vi "FABR-What Now.vi"(0 "Runtime in":T1, 2 "Queue in":refnum<queue>, 7 "SCL in":cluster{T3[]}[](array[cluster]), 11 "error in (no error)":errorcluster) -> (4 "Runtime thru":T1, 8 "SCL thru":cluster{T3[]}[](array[cluster]), 15 "error out":errorcluster)   [LabVIEW 2020]
uses:
  Typedefs/FABR-Stimulus Condition.ctl
  Typedefs/FABR-Runtime Data.ctl
  Typedefs/FABR-Stimulus Ticket.ctl
  Typedefs/FABR-Queue Data.ctl
  Typedefs/FABR-Parameters.ctl
  Typedefs/FABR-Stimulus.ctl
  Typedefs/FABR-Sequence.ctl
  Typedefs/FABR-Order.ctl
  Typedefs/FABR-Response.ctl
  Threshold Estimation VIs/ABR3-Threshold Estimation Parameters.ctl
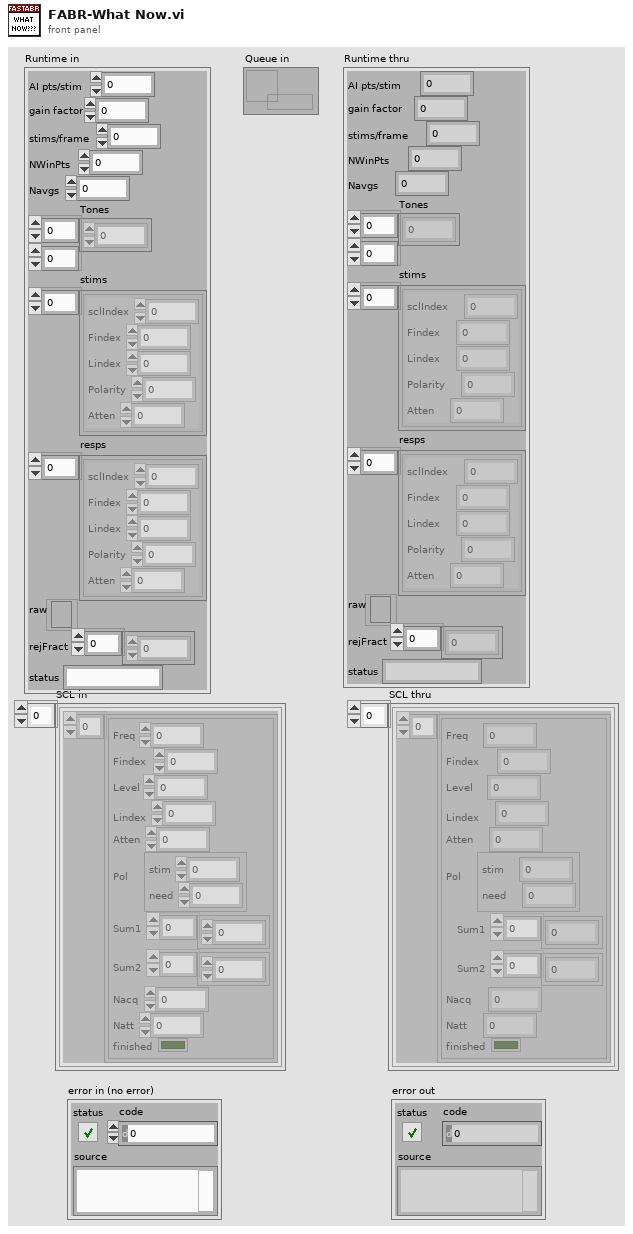
[diagram p1: front panel]
types:
  T1 = typedef "FABR-Runtime Data.ctl" = cluster{"AI pts/stim":i32, "gain factor":dbl, "stims/frame":i32, "NWinPts":i32, "Navgs":i32, "Tones":dbl[][], "stims":T2[], "resps":T2[], "raw":refnum<file>, "rejFract":dbl[], "status":string}
  T2 = typedef "FABR-Stimulus Ticket.ctl" = cluster{"sclIndex":i32, "Findex":i32, "Lindex":i32, "Polarity":i32, "Atten":dbl}
  T3 = typedef "FABR-Stimulus Condition.ctl" = cluster{"Freq":dbl, "Findex":i32, "Level":dbl, "Lindex":i32, "Atten":dbl, "Pol":cluster{"stim":i32, "need":i32}, "Sum1":dbl[], "Sum2":dbl[], "Nacq":i32, "Natt":i32, "finished":bool}
  T4 = typedef "FABR-Queue Data.ctl" = cluster{"Action":string, "Path":path, "Params":T5, "Threshold":T10, "error":errorcluster}
  T5 = typedef "FABR-Parameters.ctl" = cluster{"Stimulus":T6, "Sequence":T7, "Response":T9, "Reject":dbl}
  T6 = typedef "FABR-Stimulus.ctl" = cluster{"Destination":string, "Rep rate (/sec)":dbl, "Alternate Polarity":bool, "Duration (ms)":dbl, "Ramp (ms)":dbl, "Fs (Hz)":dbl, "Frame size (s)":dbl}
  T7 = typedef "FABR-Sequence.ctl" = cluster{"Freq":cluster{"Start (kHz)":dbl, "Stop (kHz)":dbl, "Step (oct)":dbl, "Skip (oct)":dbl}, "Level":cluster{"Start (dB)":i32, "Stop (dB)":i32, "Step (dB)":i32}, "Order":T8}
  T8 = typedef "FABR-Order.ctl" = enum16{"Interleaved"}
  T9 = typedef "FABR-Response.ctl" = cluster{"Gain":dbl, "Averages":i32, "Window (ms)":sgl, "Fs (Hz)":dbl, "Save raw":bool}
  T10 = typedef "ABR3-Threshold Estimation Parameters.ctl" = cluster{"Tmin (ms)":dbl, "Tmax (ms)":dbl, "CC criterion":dbl, "adjR2 criterion":dbl}
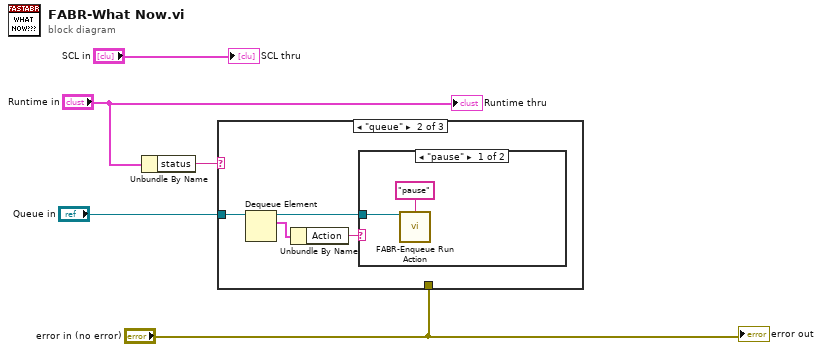
[diagram p0: block diagram]
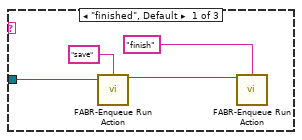
[diagram p2: hidden frame]
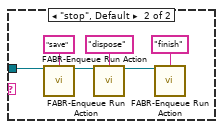
[diagram p3: hidden frame]
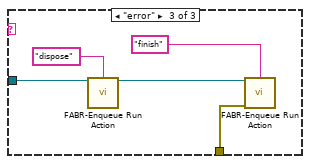
[diagram p4: hidden frame]
diagram:
  n1 = Unbundle By Name("Runtime in") -> ("status"=w3:string)
  n2 = case shown="\"queue\"" w3 {
    tunnel: "Queue in" -> [w9 w13 w25]
    tunnel: "error in (no error)" -> [_ _ w22]
    frame "finished", Default {
      n3 = call "FABR-Enqueue Run Action.vi"("Run queue"=w9, "Action"="save") -> ("queue out"=w6:refnum<queue>)  [unwired: 13 in]
      n4 = call "FABR-Enqueue Run Action.vi"("Run queue"=w6, "Action"="finish") -> ()  [unwired: 13 in, 1 out]
    }
    frame "queue" {
      n5 = Dequeue Element(queue=w13) -> (queue out=w10:refnum<queue>, element=w12:T4)  [unwired: 2 in, 2 out]
      n6 = Unbundle By Name(w12) -> ("Action"=w11:string)
      n7 = case shown="\"pause\"" w11 {
        tunnel: w10 -> [w14 w20]
        frame "pause" {
          n8 = call "FABR-Enqueue Run Action.vi"("Run queue"=w14, "Action"="pause") -> ()  [unwired: 13 in, 1 out]
        }
        frame "stop", Default {
          n9 = call "FABR-Enqueue Run Action.vi"("Run queue"=w20, "Action"="save") -> ("queue out"=w18:refnum<queue>)  [unwired: 13 in]
          n10 = call "FABR-Enqueue Run Action.vi"("Run queue"=w18, "Action"="dispose") -> ("queue out"=w16:refnum<queue>)  [unwired: 13 in]
          n11 = call "FABR-Enqueue Run Action.vi"("Run queue"=w16, "Action"="finish") -> ()  [unwired: 13 in, 1 out]
        }
      }
    }
    frame "error" {
      n12 = call "FABR-Enqueue Run Action.vi"("Run queue"=w25, "Action"="dispose") -> ("queue out"=w23:refnum<queue>)  [unwired: 13 in]
      n13 = call "FABR-Enqueue Run Action.vi"("Run queue"=w23, "Action"="finish", "error"=w22) -> ()  [unwired: 12 in, 1 out]
    }
  }
  "SCL thru" <- "SCL in"
  "Runtime thru" <- "Runtime in"
  "error out" <- "error in (no error)"
